vi "endEventToString.vi"(8 "error in (no error)":errorcluster, 11 "SingleToneRamp in":refnum<class "SingleToneRamp.lvclass">) -> (0 "error out":errorcluster, 2 "eventStringArray":string[](array[string]), 3 "SingleToneRamp out":refnum<class "SingleToneRamp.lvclass">)   [LabVIEW 2009, in "Tools.lvlib" / "Scripting.lvlib" / "SingleToneRamp.lvclass"]
uses:
  SingleToneRamp.lvclass
  ScriptEvent.lvclass
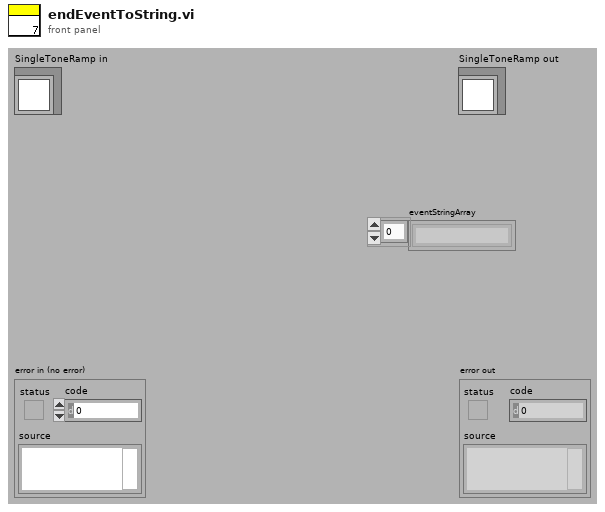
[diagram p1: front panel]
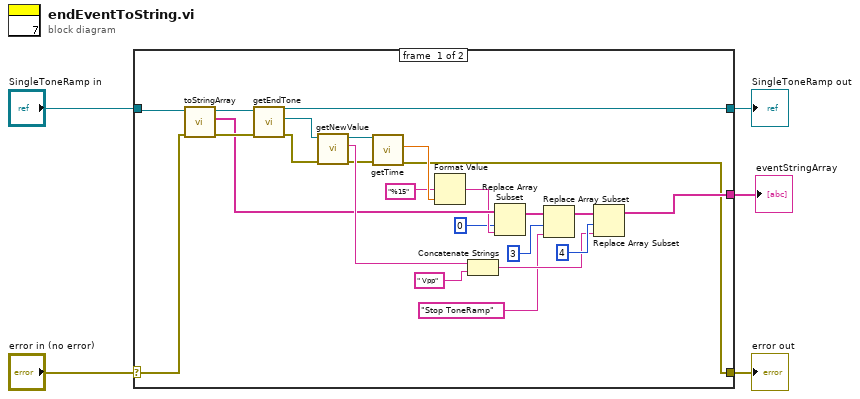
[diagram p0: block diagram]
diagram:
  n1 = case shown="No Error" "error in (no error)" {
    selector: "error in (no error)" -> [w28 w31]
    tunnel: [w6 w31] -> w4
    tunnel: [w18 w30] -> w2
    tunnel: "SingleToneRamp in" -> [w29 w30]
    tunnel: [w19 _] -> w1
    frame #0 {
      n2 = call-dynamic "toStringArray.vi"("error in (no error)"=w28, "SingleToneRamp in"=w29) -> ("error out"=w25:errorcluster, "eventStringArray"=w17:string[], "SingleToneRamp out"=w27:refnum<class "SingleToneRamp.lvclass">)  [unwired: 7 in]
      n3 = call "getEndTone.vi"("error in (no error)"=w25, "SingleToneRamp.lvclass in"=w27) -> ("error out"=w24:errorcluster, "endTone"=w26:refnum<class "SingleTone.lvclass">, "SingleToneRamp.lvclass out"=w18:refnum<class "SingleToneRamp.lvclass">)  [unwired: 7 in]
      n4 = call "getNewValue.vi"("error in (no error)"=w24, "ScriptEvent.lvclass in"=w26) -> ("error out"=w15:errorcluster, "newValue"=w22:string, "ScriptEvent.lvclass out"=w16:refnum<class "SingleTone.lvclass">)  [unwired: 7 in]
      n5 = call "getTime.vi"("error in (no error)"=w15, "ScriptEvent.lvclass in"=w16) -> ("error out"=w6:errorcluster, "time"=w14:dbl)  [unwired: 7 in, 1 out]
      n6 = Format Value(format string="%15", value (0)=w14) -> (output string=w12:string)  [unwired: 1 in]
      n7 = Concatenate Strings(w22, " Vpp") -> (w20:string)
      n8 = Replace Array Subset(array=w17, new element=w12, index=0) -> (w10:string[])
      n9 = Replace Array Subset(array=w10, new element="Stop ToneRamp", index=3) -> (w7:string[])
      n10 = Replace Array Subset(array=w7, new element=w20, index=4) -> (w19:string[])
    }
    frame #1 {
    }
  }
  "error out" <- w4
  "SingleToneRamp out" <- w2
  "eventStringArray" <- w1
